vi "Path Direction Select.vi"(7 "Danger":bool, 9 "Target Direction":T1, 11 "Position ID":T2) -> (3 "Direction Array":T1[](array[typedef]))   [LabVIEW 2017, in "AntFarm_MB.lvclass"]
uses:
  AntFarm_MB.lvclass
  Type Defs/Direction Enum.ctl
  TypeDefs/ENUM_Position ID.ctl
  Type Defs/SB Type Defs.lvlib
panel:
  out "Seconday Move Direction Out":T1
  out "Primary Move Direction Out":T1
  out "Primary Queen Direction Out":T1
  out "Secondary Queen Direction Out":T1
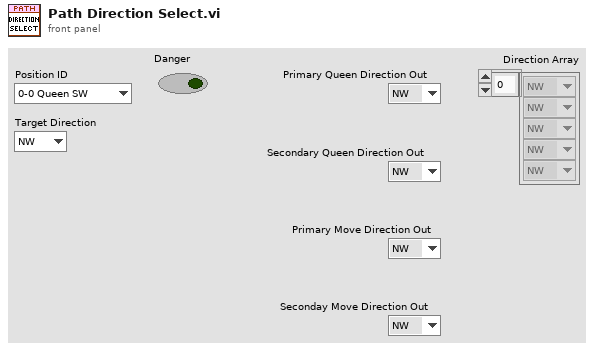
[diagram p1: front panel]
types:
  T1 = typedef "SB Type Defs.lvlib/Direction Enum.ctl" = enum16{"NW", "N", "NE", "E", "SE", "S", "SW", "W"}
  T2 = typedef "ENUM_Position ID.ctl" = enum16{"0-0 Queen SW", "0-1 Path E", "0-2 Queen NW", "0-3 Path W", "1-0 Path S", "1-1 Larva SW", "1-2 Path N", "1-3 Larva NW", "2-0 Queen SE", "2-1 Path W", "2-2 Queen NE", "2-3 Path E", "3-0 Path N", "3-1 Larva SE", "3-2 Path S", "3-3 Larva NE"}
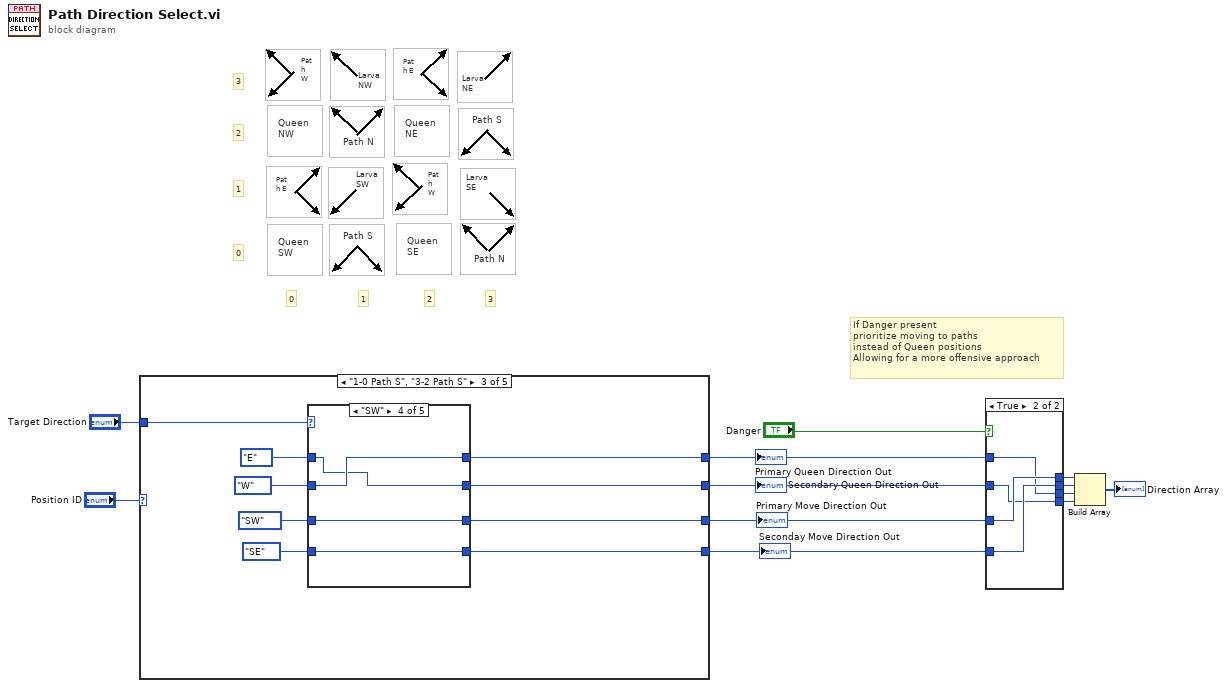
[diagram p0: block diagram]
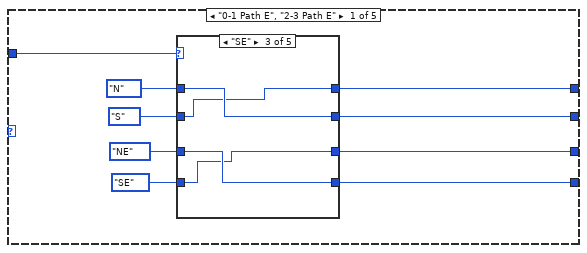
[diagram p3: hidden frame]
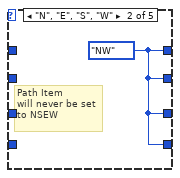
[diagram p5: hidden frame]
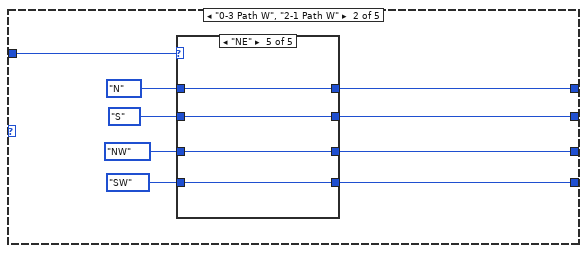
[diagram p8: hidden frame]
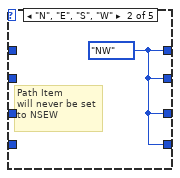
[diagram p10: hidden frame]
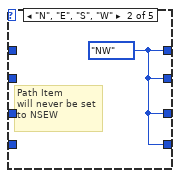
[diagram p14: hidden frame]
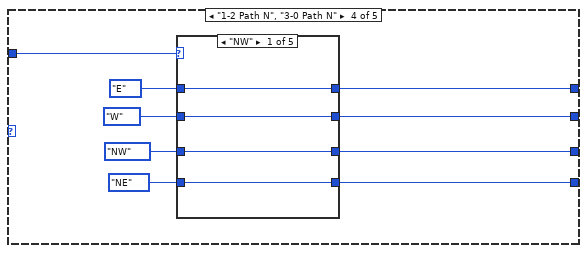
[diagram p17: hidden frame]
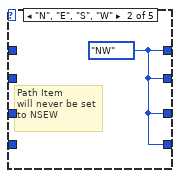
[diagram p18: hidden frame]
diagram:
  # "Path N"
  # "Path E"
  # "Path S"
  # "Path W"
  # "Path W"
  # "Path S"
  # "Path E"
  # "Path N"
  # "Larva\nNE"
  # "Larva\nSW"
  # "Larva\nNW"
  # "Queen\nNW"
  # "Queen\nNE"
  # "Queen\nSE"
  # "Larva\nSE"
  # "3"
  # "2"
  # "1"
  # "0"
  # "3"
  # "2"
  # "1"
  # "0"
  # "Queen\nSW"
  # "If Danger present\nprioritize moving to paths\ninstead of Queen positions\nAllowing for a more offensive approach"
  n1 = case shown="\"1-0 Path S\", \"3-2 Path S\"" "Position ID" {
    tunnel: "Target Direction" -> [w21 w47 w73 w99 _]
    tunnel: [w20 w46 w72 w98 w117] -> w5
    tunnel: [w19 w45 w71 w97 w117] -> w8
    tunnel: [w18 w44 w70 w96 w117] -> w4
    tunnel: [w17 w43 w69 w95 w117] -> w2
    frame "0-1 Path E", "2-3 Path E" {
      n2 = case shown="\"SE\"" w21 {
        tunnel: [w25 w26 w29 w34 w38] -> w19
        tunnel: [w24 w26 w30 w33 w37] -> w20
        tunnel: [w23 w26 w27 w32 w36] -> w18
        tunnel: [w22 w26 w28 w31 w35] -> w17
        tunnel: Direction_Enum."N" ("Primary Direction") -> [w25 _ w30 w33 w38]
        tunnel: Direction_Enum."S" ("Primary Direction") -> [w24 _ w29 w34 w37]
        tunnel: Direction_Enum."NE" ("Primary Direction") -> [w23 _ w28 w31 w36]
        tunnel: Direction_Enum."SE" ("Primary Direction") -> [w22 _ w27 w32 w35]
        frame "NW" {
        }
        frame "N", "E", "S", "W" {
          w26 = Direction_Enum."NW" ("Primary Direction")
          # "Path Item\nwill never be set\nto NSEW"
        }
        frame "SE" {
        }
        frame "SW" {
        }
        frame "NE" {
        }
      }
    }
    frame "0-3 Path W", "2-1 Path W" {
      n3 = case shown="\"NE\"" w47 {
        tunnel: [w51 w52 w55 w60 w64] -> w45
        tunnel: [w50 w52 w56 w59 w63] -> w46
        tunnel: [w49 w52 w53 w58 w62] -> w44
        tunnel: [w48 w52 w54 w57 w61] -> w43
        tunnel: Direction_Enum."N" ("Primary Direction") -> [w51 _ w56 w59 w64]
        tunnel: Direction_Enum."S" ("Primary Direction") -> [w50 _ w55 w60 w63]
        tunnel: Direction_Enum."NW" ("Primary Direction") -> [w49 _ w54 w57 w62]
        tunnel: Direction_Enum."SW" ("Primary Direction") -> [w48 _ w53 w58 w61]
        frame "NW" {
        }
        frame "N", "E", "S", "W" {
          w52 = Direction_Enum."NW" ("Primary Direction")
          # "Path Item\nwill never be set\nto NSEW"
        }
        frame "SE" {
        }
        frame "SW" {
        }
        frame "NE" {
        }
      }
    }
    frame "1-0 Path S", "3-2 Path S" {
      n4 = case shown="\"SW\"" w73 {
        tunnel: [w77 w78 w81 w86 w90] -> w71
        tunnel: [w76 w78 w82 w85 w89] -> w72
        tunnel: [w75 w78 w79 w84 w88] -> w70
        tunnel: [w74 w78 w80 w83 w87] -> w69
        tunnel: Direction_Enum."E" ("Primary Direction") -> [w77 _ w82 w85 w90]
        tunnel: Direction_Enum."W" ("Primary Direction") -> [w76 _ w81 w86 w89]
        tunnel: Direction_Enum."SW" ("Primary Direction") -> [w75 _ w80 w84 w87]
        tunnel: Direction_Enum."SE" ("Primary Direction") -> [w74 _ w79 w83 w88]
        frame "NW" {
        }
        frame "N", "E", "S", "W" {
          w78 = Direction_Enum."NW" ("Primary Direction")
          # "Path Item\nwill never be set\nto NSEW"
        }
        frame "SE" {
        }
        frame "SW" {
        }
        frame "NE" {
        }
      }
    }
    frame "1-2 Path N", "3-0 Path N" {
      n5 = case shown="\"NW\"" w99 {
        tunnel: [w103 w104 w107 w112 w116] -> w97
        tunnel: [w102 w104 w108 w111 w115] -> w98
        tunnel: [w101 w104 w105 w110 w114] -> w96
        tunnel: [w100 w104 w106 w109 w113] -> w95
        tunnel: Direction_Enum."E" ("Primary Direction") -> [w103 _ w108 w111 w116]
        tunnel: Direction_Enum."W" ("Primary Direction") -> [w102 _ w107 w112 w115]
        tunnel: Direction_Enum."NW" ("Primary Direction") -> [w101 _ w106 w110 w113]
        tunnel: Direction_Enum."NE" ("Primary Direction") -> [w100 _ w105 w109 w114]
        frame "NW" {
        }
        frame "N", "E", "S", "W" {
          w104 = Direction_Enum."NW" ("Primary Direction")
          # "Path Item\nwill never be set\nto NSEW"
        }
        frame "SE" {
        }
        frame "SW" {
        }
        frame "NE" {
        }
      }
    }
    frame Default {
      w117 = Direction_Enum."NW" ("Primary Direction")
      # "This vi is only\nfor path cases"
    }
  }
  "Secondary Queen Direction Out" <- w5
  "Primary Queen Direction Out" <- w8
  "Primary Move Direction Out" <- w4
  "Seconday Move Direction Out" <- w2
  n6 = case shown="True" "Danger" {
    tunnel: w8 -> [w121 w123]
    tunnel: [w121 w125] -> w7
    tunnel: w5 -> [w120 w122]
    tunnel: [w120 w124] -> w6
    tunnel: w4 -> [w119 w125]
    tunnel: [w119 w123] -> w3
    tunnel: w2 -> [w118 w124]
    tunnel: [w118 w122] -> w1
    frame False {
    }
    frame True {
    }
  }
  n7 = Build Array(w7, w6, w3, w1) -> (→"Direction Array":T1[])
